vi "Bounds.vi"(1 "XRef":refnum<vi>, 2 "State In":T2={"Input Type"=variant(dbl 0.0), "Selection"=0, "Element Names"=[], "Type Strings"=[], "Element Types"=[]}) -> (0 "Bounds":cluster{"Width":T1, "Height":T1})   [LabVIEW 2015, in "Construct-Tagged-Union.xnode"]
doc: "This ability VI is used to tell LabVIEW your current bounds. If you want to update your bounds, you must inform LabVIEW through the UpdateImageAndBounds reply of another ability VI. If you change your bounds, you will also probably want to update your image.\n\nDefault behavior: None.\n\nThis ability does not provide UI and OS messages are not handled."
uses:
  Construct-Tagged-Union.xnode
  State.ctl
  <vilib>/XNodeSupport/XNodeInt.ctl
  <vilib>/XNodeSupport/NI_XNodeSupport.lvlib
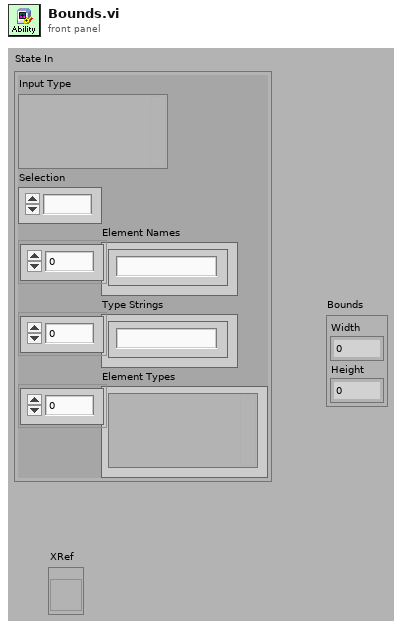
[diagram p1: front panel]
types:
  T1 = typedef "NI_XNodeSupport.lvlib/XNodeInt.ctl" = i32
  T2 = typedef "Construct-Tagged-Union.xnode/State.ctl" = cluster{"Input Type":variant, "Selection":i32, "Element Names":string[], "Type Strings":string[], "Element Types":variant[]}
  T3 = cluster{"left":i16, "top":i16, "right":i16, "bottom":i16}
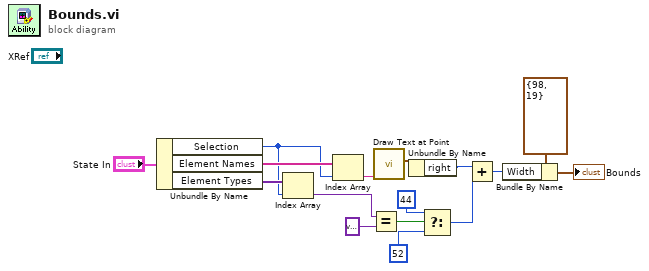
[diagram p0: block diagram]
diagram:
  n1 = Unbundle By Name("State In") -> ("Selection"=w7:i32, "Element Names"=w13:string[], "Element Types"=w8:variant[])
  n2 = Index Array(array=w8, index=w7) -> (element=w6:variant)
  n3 = Index Array(array=w13, index=w7) -> (element=w12:string)
  n4 = Equal?(x=w6, y=variant) -> (x = y?=w4:bool)
  n5 = call <vilib>:"Draw Text at Point.vi"("text"=w12) -> ("text rect"=w11:T3)  [unwired: 9 in, 1 out]
  n6 = Unbundle By Name(w11) -> ("right"=w10:i16)
  n7 = Select(t=i16 44 ("x"), s=w4, f=i16 52 ("x")) -> (s? t:f=w1:i16)
  n8 = Add(x=w10, y=w1) -> (x+y=w9:i16)
  n9 = Bundle By Name(cluster=cluster{"Width":T1, "Height":T1} {"Width"=98, "Height"=19} ("Bounds"), "Width"=w9) -> (→"Bounds":cluster{"Width":T1, "Height":T1})
